vi "Car Data.vi"(1 "file path (dialog if empty)":path) -> (0 "CAR DATA":T1)   [LabVIEW 2014]
uses:
  Type Def/CAN Message.ctl
  Type Def/CAR Data Cluster.ctl
  <vilib>/Utility/file.llb/Read From Spreadsheet File (string).vi
panel:
  out "Time Size":i32
  out "number of rows":i32
  out "Time":dbl[](array[numeric]) format="%.2f"
  out "Array":T2[](array[typedef])
  out "DECAYIGN(+) - DECAYIGN(-)":dbl
  out "DECAYINJ(+) - DECAYINJ(-)":dbl
  out "DTPS-":dbl
  out "DTPS+":dbl
  out "Speed 2":dbl
  out "Speed 1":dbl
  out "Phase High":dbl
  out "Phase Low":dbl
  out "Spark 1":dbl
  out "Inj Low":dbl
  out "K Lambda 2":dbl
  out "K Lambda 1":dbl
  out "Lambda 2 AVG":dbl
  out "Lambda 2 RAW":dbl
  out "Lambda 1 RAW":dbl
  out "Lambda 1 AVG":dbl
  out "BAR0":u32
  out "VBB 3":dbl
  out "VBB 2":dbl
  out "VBB 1":dbl
  out "T Oil":u32
  out "T Air":i32
  out "T H20":i32
  out "map":u32
  out "TPS":dbl
  out "rev/min":u32
  out "revs":u32
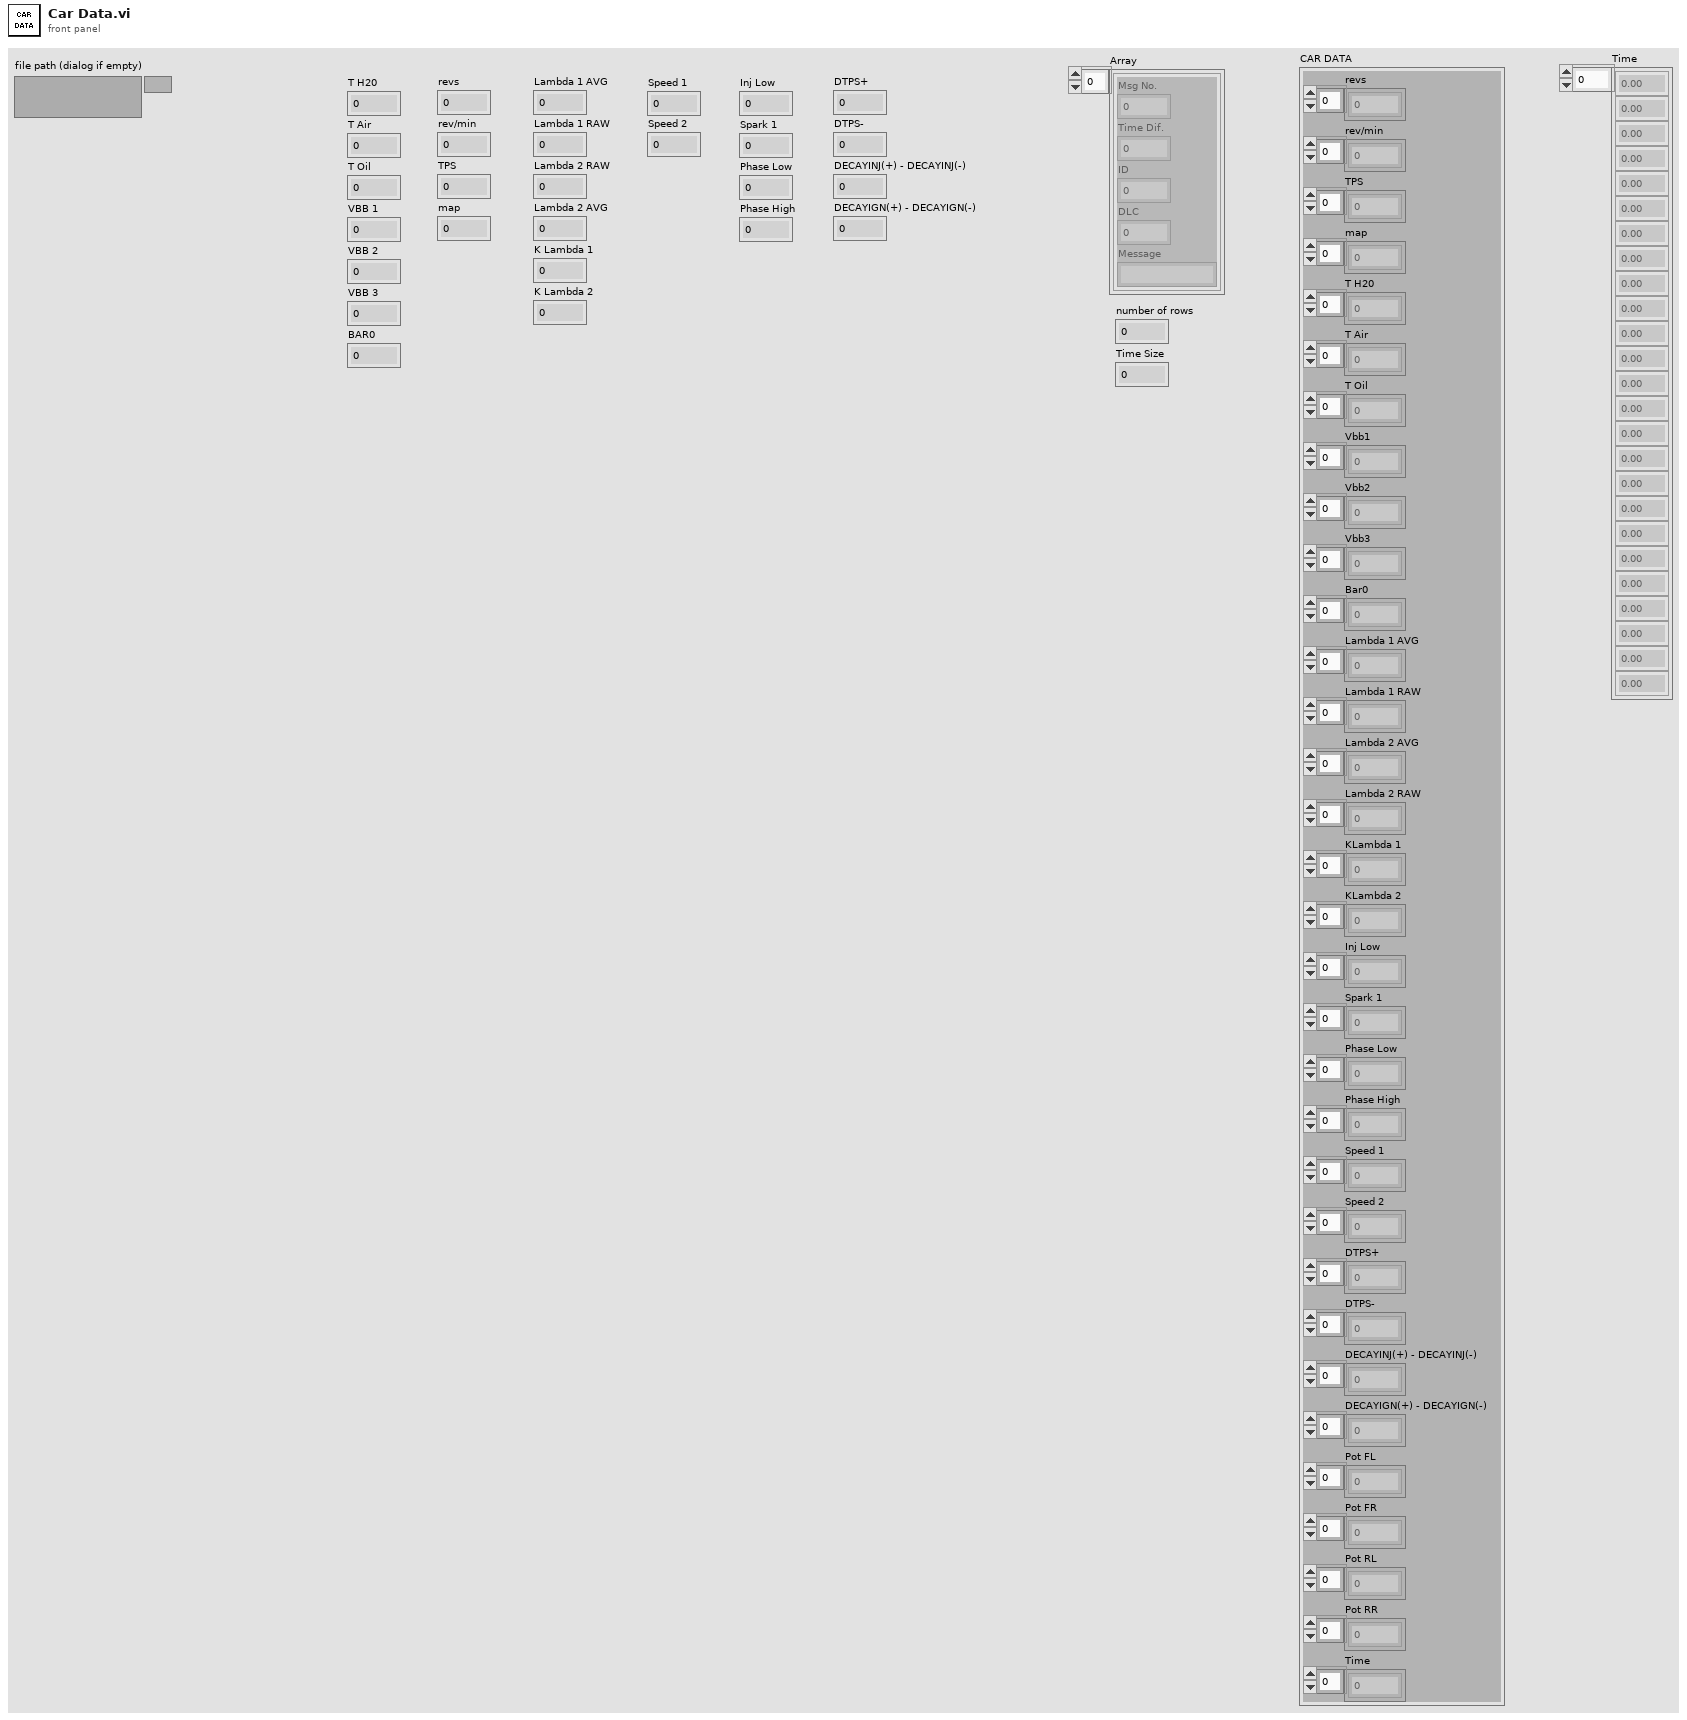
[diagram p1: front panel]
types:
  T1 = typedef "CAR Data Cluster.ctl" = cluster{"revs":dbl[], "rev/min":dbl[], "TPS":dbl[], "map":dbl[], "T H20":dbl[], "T Air":dbl[], "T Oil":dbl[], "Vbb1":dbl[], "Vbb2":dbl[], "Vbb3":dbl[], "Bar0":dbl[], "Lambda 1 AVG":dbl[], "Lambda 1 RAW":dbl[], "Lambda 2 AVG":dbl[], "Lambda 2 RAW":dbl[], "KLambda 1":dbl[], "KLambda 2":dbl[], "Inj Low":dbl[], "Spark 1":dbl[], "Phase Low":dbl[], "Phase High":dbl[], "Speed 1":dbl[], "Speed 2":dbl[], "DTPS+":dbl[], "DTPS-":dbl[], "DECAYINJ(+) - DECAYINJ(-)":dbl[], "DECAYIGN(+) - DECAYIGN(-)":dbl[], "Pot FL":dbl[], "Pot FR":dbl[], "Pot RL":dbl[], "Pot RR":dbl[], "Time":dbl[]}
  T2 = typedef "CAN Message.ctl" = cluster{"Msg No.":i32, "Time Dif.":i32, "ID":i32, "DLC":i32, "Message":string}
  T3 = cluster{"revs":dbl[], "rev/min":dbl[], "TPS":dbl[], "map":dbl[], "T H20":dbl[], "T Air":dbl[], "T Oil":dbl[], "Vbb1":dbl[], "Vbb2":dbl[], "Vbb3":dbl[], "Bar0":dbl[], "Lambda 1 AVG":dbl[], "Lambda 1 RAW":dbl[], "Lambda 2 AVG":dbl[], "Lambda 2 RAW":dbl[], "KLambda 1":dbl[], "KLambda 2":dbl[], "Inj Low":dbl[], "Spark 1":dbl[], "Phase Low":dbl[], "Phase High":dbl[], "Speed 1":dbl[], "Speed 2":dbl[], "DTPS+":dbl[], "DTPS-":dbl[], "DECAYINJ(+) - DECAYINJ(-)":dbl[], "DECAYIGN(+) - DECAYIGN(-)":dbl[], "Pot FL":dbl[], "Pot FR":dbl[], "Pot RL":dbl[], "Pot RR":dbl[], "Time":dbl[]}
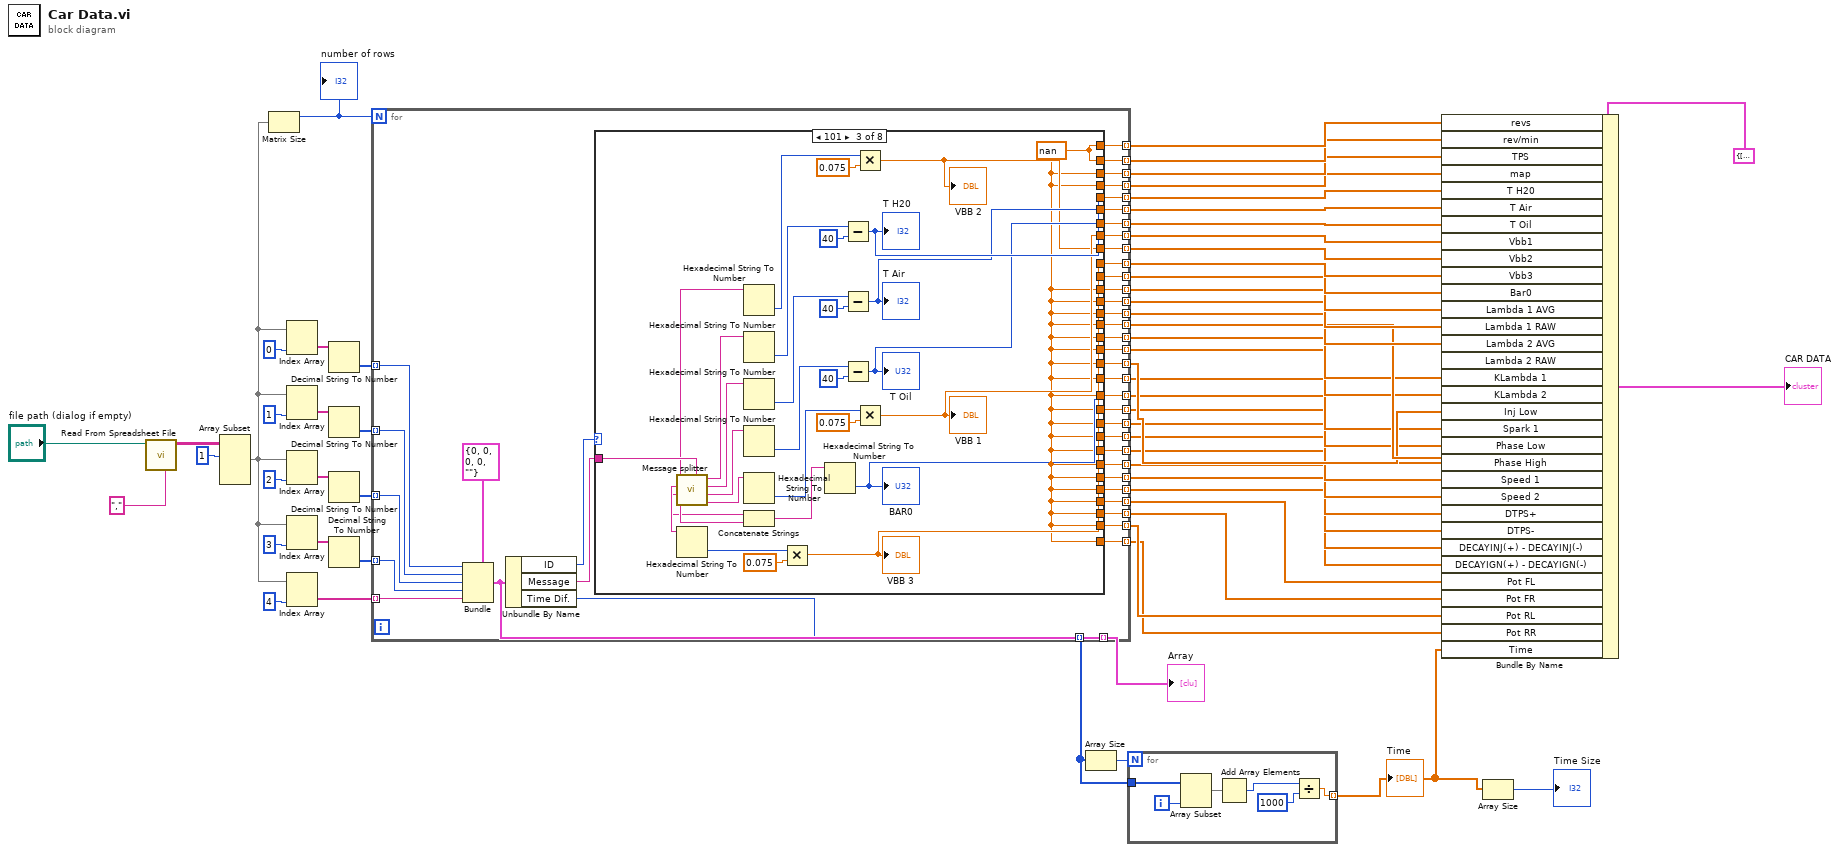
[diagram p0: block diagram]
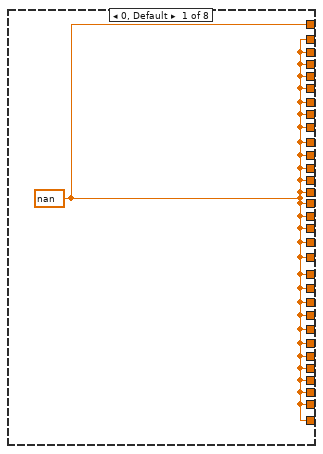
[diagram p2: hidden frame]
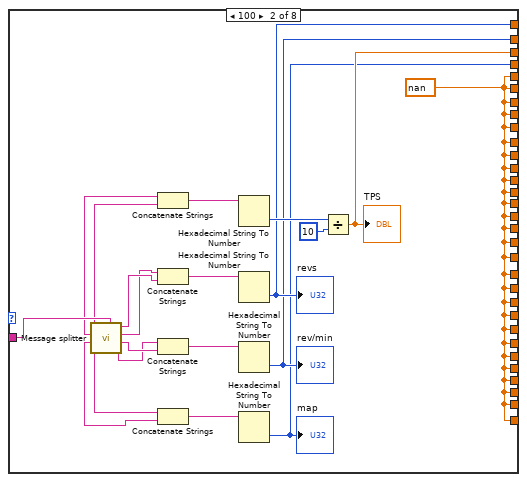
[diagram p3: hidden frame]
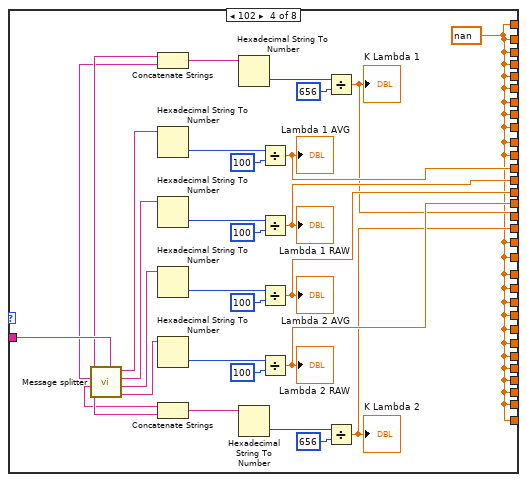
[diagram p4: hidden frame]
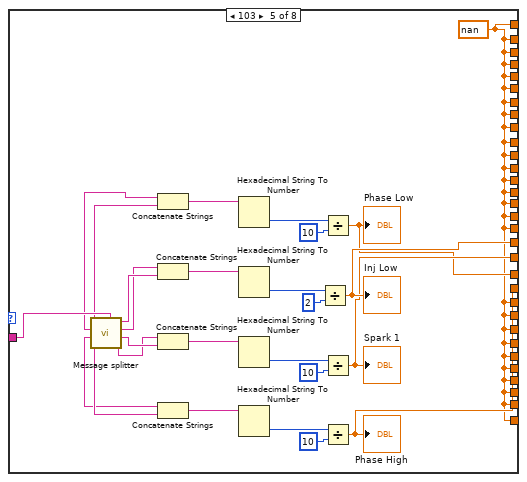
[diagram p5: hidden frame]
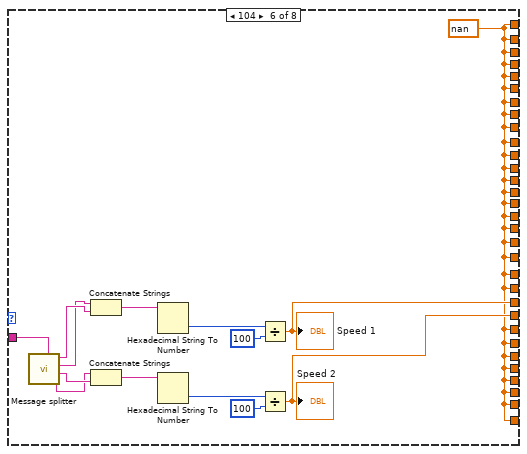
[diagram p6: hidden frame]
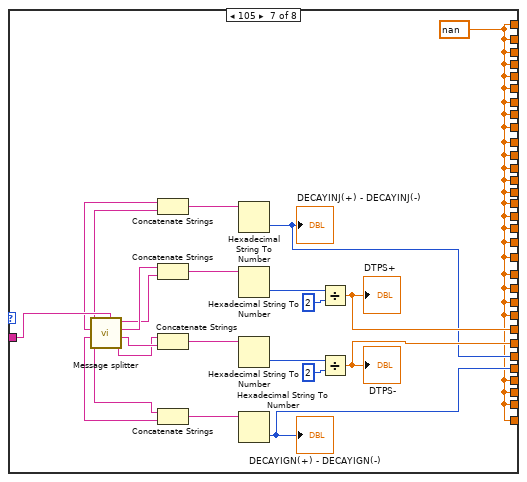
[diagram p7: hidden frame]
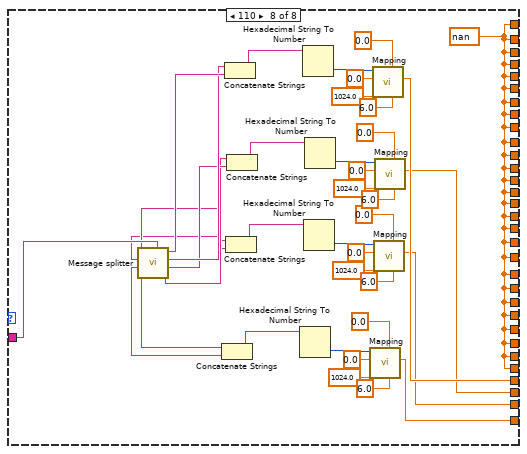
[diagram p8: hidden frame]
diagram:
  n1 = call-poly <vilib>:"Read From Spreadsheet File.vi"("delimiter (\\t)"="," ("delimiter (\\t)"), "file path (dialog if empty)"="file path (dialog if empty)") -> ("all rows"=w40:string[][])  [unwired: 5 in, 4 out]
  n2 = Array Subset(array=w40, index (row)=1 ("index")) -> (w51:string[][])  [unwired: 3 in]
  n3 = Matrix Size(0:w51) -> (1:w56:i32)  [unwired: 1 out]
  "number of rows" <- w56
  n4 = Index Array(array=w51, index (col)=0 ("index")) -> (element=w45:string[])  [unwired: 1 in]
  n5 = Index Array(array=w51, index (col)=1 ("index")) -> (element=w44:string[])  [unwired: 1 in]
  n6 = Index Array(array=w51, index (col)=2 ("index")) -> (element=w43:string[])  [unwired: 1 in]
  n7 = Index Array(array=w51, index (col)=3 ("index")) -> (element=w42:string[])  [unwired: 1 in]
  n8 = Index Array(array=w51, index (col)=4 ("index")) -> (element=w41:string[])  [unwired: 1 in]
  n9 = Decimal String To Number(string=w45) -> (number=w55:i32[])  [unwired: 2 in, 1 out]
  n10 = Decimal String To Number(string=w44) -> (number=w54:i32[])  [unwired: 2 in, 1 out]
  n11 = Decimal String To Number(string=w43) -> (number=w53:i32[])  [unwired: 2 in, 1 out]
  n12 = Decimal String To Number(string=w42) -> (number=w52:i32[])  [unwired: 2 in, 1 out]
  n13 = for {
    N: w56 -> [_]
    tunnel: w55 -> [w98] mode=indexing
    tunnel: w54 -> [w97] mode=indexing
    tunnel: w53 -> [w96] mode=indexing
    tunnel: w52 -> [w95] mode=indexing
    tunnel: [w93] -> w37 mode=indexing
    tunnel: w41 -> [w94] mode=indexing
    tunnel: [w90] -> w39 mode=indexing
    tunnel: [w89] -> w33 mode=indexing
    tunnel: [w88] -> w35 mode=indexing
    tunnel: [w87] -> w34 mode=indexing
    tunnel: [w86] -> w32 mode=indexing
    tunnel: [w85] -> w31 mode=indexing
    tunnel: [w84] -> w30 mode=indexing
    tunnel: [w83] -> w29 mode=indexing
    tunnel: [w82] -> w28 mode=indexing
    tunnel: [w81] -> w27 mode=indexing
    tunnel: [w80] -> w26 mode=indexing
    tunnel: [w79] -> w25 mode=indexing
    tunnel: [w78] -> w24 mode=indexing
    tunnel: [w77] -> w23 mode=indexing
    tunnel: [w76] -> w22 mode=indexing
    tunnel: [w75] -> w21 mode=indexing
    tunnel: [w74] -> w20 mode=indexing
    tunnel: [w73] -> w19 mode=indexing
    tunnel: [w72] -> w18 mode=indexing
    tunnel: [w71] -> w17 mode=indexing
    tunnel: [w70] -> w16 mode=indexing
    tunnel: [w69] -> w15 mode=indexing
    tunnel: [w68] -> w14 mode=indexing
    tunnel: [w67] -> w13 mode=indexing
    tunnel: [w66] -> w12 mode=indexing
    tunnel: [w65] -> w11 mode=indexing
    tunnel: [w64] -> w10 mode=indexing
    tunnel: [w63] -> w9 mode=indexing
    tunnel: [w62] -> w7 mode=indexing
    tunnel: [w61] -> w6 mode=indexing
    tunnel: [w60] -> w5 mode=indexing
    tunnel: [w59] -> w4 mode=indexing
    n14 = Bundle(cluster=T2 {"Msg No."=0, "Time Dif."=0, "ID"=0, "DLC"=0, "Message"=""}, "Msg No."=w98, "Time Dif."=w97, "ID"=w96, "DLC"=w95, "Message"=w94) -> (w93:T2)
    n15 = Unbundle By Name(w93) -> ("ID"=w92:i32, "Message"=w91:string, "Time Dif."=w90:i32)
    n16 = case shown="101" w92 {
      tunnel: w91 -> [_ w114 w137 w180 w206 w220 w242 w280]
      tunnel: [w100 w113 w121 w151 w181 w207 w221 w279] -> w89
      tunnel: [w100 w112 w121 w151 w181 w207 w221 w279] -> w88
      tunnel: [w100 w111 w121 w151 w181 w207 w221 w279] -> w87
      tunnel: [w100 w110 w121 w151 w181 w207 w221 w279] -> w86
      tunnel: [w100 w101 w130 w151 w181 w207 w221 w279] -> w85
      tunnel: [w100 w101 w129 w151 w181 w207 w221 w279] -> w84
      tunnel: [w100 w101 w128 w151 w181 w207 w221 w279] -> w83
      tunnel: [w100 w101 w127 w151 w181 w207 w221 w279] -> w82
      tunnel: [w100 w101 w126 w151 w181 w207 w221 w279] -> w81
      tunnel: [w100 w101 w125 w151 w181 w207 w221 w279] -> w80
      tunnel: [w100 w101 w124 w151 w181 w207 w221 w279] -> w79
      tunnel: [w100 w101 w121 w159 w181 w207 w221 w279] -> w78
      tunnel: [w100 w101 w121 w158 w181 w207 w221 w279] -> w77
      tunnel: [w100 w101 w121 w157 w181 w207 w221 w279] -> w76
      tunnel: [w100 w101 w121 w156 w181 w207 w221 w279] -> w75
      tunnel: [w100 w101 w121 w155 w181 w207 w221 w279] -> w74
      tunnel: [w100 w101 w121 w154 w181 w207 w221 w279] -> w73
      tunnel: [w100 w101 w121 w151 w193 w207 w221 w279] -> w72
      tunnel: [w100 w101 w121 w151 w192 w207 w221 w279] -> w71
      tunnel: [w100 w101 w121 w151 w191 w207 w221 w279] -> w70
      tunnel: [w100 w101 w121 w151 w190 w207 w221 w279] -> w69
      tunnel: [w100 w101 w121 w151 w181 w213 w221 w279] -> w68
      tunnel: [w100 w101 w121 w151 w181 w212 w221 w279] -> w67
      tunnel: [w100 w101 w121 w151 w181 w207 w233 w279] -> w66
      tunnel: [w100 w101 w121 w151 w181 w207 w232 w279] -> w65
      tunnel: [w100 w101 w121 w151 w181 w207 w231 w279] -> w64
      tunnel: [w100 w101 w121 w151 w181 w207 w230 w279] -> w63
      tunnel: [w100 w101 w121 w151 w181 w207 w221 w270] -> w62
      tunnel: [w100 w101 w121 w151 w181 w207 w221 w261] -> w61
      tunnel: [w100 w101 w121 w151 w181 w207 w221 w244] -> w60
      tunnel: [w100 w101 w121 w151 w181 w207 w221 w243] -> w59
      frame 0, Default {
        w100 = nan
      }
      frame 100 {
        w101 = nan
        n17 = call "Message splitter.vi"("Message in"=w114) -> ("Byte 4"=w104:string, "Byte 3"=w105:string, "Byte 2"=w106:string, "Byte 1"=w107:string, "Byte 8"=w102:string, "Byte 7"=w103:string, "Byte 6"=w109:string, "Byte 5"=w108:string)  [unwired: 3 in]
        n18 = Concatenate Strings(w109, w108) -> (w118:string)
        n19 = Concatenate Strings(w106, w107) -> (w120:string)
        n20 = Concatenate Strings(w104, w105) -> (w119:string)
        n21 = Concatenate Strings(w102, w103) -> (w115:string)
        n22 = Hexadecimal String To Number(string=w118) -> (number=w117:u32)  [unwired: 2 in, 1 out]
        n23 = Hexadecimal String To Number(string=w120) -> (number=w112:u32)  [unwired: 2 in, 1 out]
        "revs" <- w112
        n24 = Hexadecimal String To Number(string=w119) -> (number=w111:u32)  [unwired: 2 in, 1 out]
        "rev/min" <- w111
        n25 = Hexadecimal String To Number(string=w115) -> (number=w110:u32)  [unwired: 2 in, 1 out]
        "map" <- w110
        n26 = Divide(x=w117, y=u32 10) -> (x/y=w113:dbl)
        "TPS" <- w113
      }
      frame 101 {
        w121 = nan
        n27 = call "Message splitter.vi"("Message in"=w137) -> ("Byte 4"=w133:string, "Byte 3"=w134:string, "Byte 2"=w135:string, "Byte 1"=w136:string, "Byte 8"=w123:string, "Byte 7"=w122:string, "Byte 6"=w131:string, "Byte 5"=w132:string)  [unwired: 3 in]
        n28 = Hexadecimal String To Number(string=w131) -> (number=w140:u32)  [unwired: 2 in, 1 out]
        n29 = Hexadecimal String To Number(string=w132) -> (number=w142:u32)  [unwired: 2 in, 1 out]
        n30 = Hexadecimal String To Number(string=w136) -> (number=w150:u32)  [unwired: 2 in, 1 out]
        n31 = Hexadecimal String To Number(string=w135) -> (number=w147:u32)  [unwired: 2 in, 1 out]
        n32 = Hexadecimal String To Number(string=w134) -> (number=w145:u32)  [unwired: 2 in, 1 out]
        n33 = Hexadecimal String To Number(string=w133) -> (number=w144:u32)  [unwired: 2 in, 1 out]
        n34 = Concatenate Strings(w122, w123) -> (w138:string)
        n35 = Multiply(x=w140, y=0.075) -> (x*y=w125:dbl)
        "VBB 3" <- w125
        n36 = Hexadecimal String To Number(string=w138) -> (number=w124:u32)  [unwired: 2 in, 1 out]
        "BAR0" <- w124
        n37 = Subtract(x=w150, y=u32 40) -> (x-y=w130:u32)
        "T H20" <- w130
        n38 = Subtract(x=w147, y=u32 40) -> (x-y=w129:u32)
        "T Air" <- w129
        n39 = Subtract(x=w145, y=u32 40) -> (x-y=w128:u32)
        "T Oil" <- w128
        n40 = Multiply(x=w142, y=0.075) -> (x*y=w126:dbl)
        "VBB 2" <- w126
        n41 = Multiply(x=w144, y=0.075) -> (x*y=w127:dbl)
        "VBB 1" <- w127
      }
      frame 102 {
        w151 = nan
        n42 = call "Message splitter.vi"("Message in"=w180) -> ("Byte 4"=w168:string, "Byte 3"=w169:string, "Byte 2"=w170:string, "Byte 1"=w179:string, "Byte 8"=w153:string, "Byte 7"=w152:string, "Byte 6"=w166:string, "Byte 5"=w167:string)  [unwired: 3 in]
        n43 = Concatenate Strings(w167, w166) -> (w163:string)
        n44 = Hexadecimal String To Number(string=w179) -> (number=w178:u32)  [unwired: 2 in, 1 out]
        n45 = Hexadecimal String To Number(string=w170) -> (number=w176:u32)  [unwired: 2 in, 1 out]
        n46 = Hexadecimal String To Number(string=w169) -> (number=w172:u32)  [unwired: 2 in, 1 out]
        n47 = Hexadecimal String To Number(string=w168) -> (number=w174:u32)  [unwired: 2 in, 1 out]
        n48 = Concatenate Strings(w152, w153) -> (w160:string)
        n49 = Hexadecimal String To Number(string=w163) -> (number=w165:u32)  [unwired: 2 in, 1 out]
        n50 = Hexadecimal String To Number(string=w160) -> (number=w162:u32)  [unwired: 2 in, 1 out]
        n51 = Divide(x=w178, y=u32 100) -> (x/y=w159:dbl)
        "Lambda 1 AVG" <- w159
        n52 = Divide(x=w176, y=u32 100) -> (x/y=w158:dbl)
        "Lambda 1 RAW" <- w158
        n53 = Divide(x=w172, y=u32 100) -> (x/y=w157:dbl)
        "Lambda 2 AVG" <- w157
        n54 = Divide(x=w174, y=u32 100) -> (x/y=w156:dbl)
        "Lambda 2 RAW" <- w156
        n55 = Divide(x=w165, y=u32 656) -> (x/y=w155:dbl)
        "K Lambda 1" <- w155
        n56 = Divide(x=w162, y=u32 656) -> (x/y=w154:dbl)
        "K Lambda 2" <- w154
      }
      frame 103 {
        w181 = nan
        n57 = call "Message splitter.vi"("Message in"=w206) -> ("Byte 4"=w186:string, "Byte 3"=w187:string, "Byte 2"=w188:string, "Byte 1"=w189:string, "Byte 8"=w183:string, "Byte 7"=w182:string, "Byte 6"=w185:string, "Byte 5"=w184:string)  [unwired: 3 in]
        n58 = Concatenate Strings(w185, w184) -> (w199:string)
        n59 = Concatenate Strings(w188, w189) -> (w205:string)
        n60 = Concatenate Strings(w186, w187) -> (w202:string)
        n61 = Concatenate Strings(w182, w183) -> (w196:string)
        n62 = Hexadecimal String To Number(string=w199) -> (number=w198:u32)  [unwired: 2 in, 1 out]
        n63 = Hexadecimal String To Number(string=w205) -> (number=w204:u32)  [unwired: 2 in, 1 out]
        n64 = Hexadecimal String To Number(string=w202) -> (number=w201:u32)  [unwired: 2 in, 1 out]
        n65 = Hexadecimal String To Number(string=w196) -> (number=w195:u32)  [unwired: 2 in, 1 out]
        n66 = Divide(x=w204, y=u32 2) -> (x/y=w193:dbl)
        "Inj Low" <- w193
        n67 = Divide(x=w198, y=u32 10) -> (x/y=w191:dbl)
        "Phase Low" <- w191
        n68 = Divide(x=w201, y=u32 10) -> (x/y=w192:dbl)
        "Spark 1" <- w192
        n69 = Divide(x=w195, y=u32 10) -> (x/y=w190:dbl)
        "Phase High" <- w190
      }
      frame 104 {
        w207 = nan
        n70 = call "Message splitter.vi"("Message in"=w220) -> ("Byte 4"=w208:string, "Byte 3"=w209:string, "Byte 2"=w210:string, "Byte 1"=w211:string)  [unwired: 3 in, 4 out]
        n71 = Concatenate Strings(w210, w211) -> (w219:string)
        n72 = Concatenate Strings(w208, w209) -> (w214:string)
        n73 = Hexadecimal String To Number(string=w219) -> (number=w218:u32)  [unwired: 2 in, 1 out]
        n74 = Hexadecimal String To Number(string=w214) -> (number=w216:u32)  [unwired: 2 in, 1 out]
        n75 = Divide(x=w218, y=u32 100) -> (x/y=w213:dbl)
        "Speed 1" <- w213
        n76 = Divide(x=w216, y=u32 100) -> (x/y=w212:dbl)
        "Speed 2" <- w212
      }
      frame 105 {
        w221 = nan
        n77 = call "Message splitter.vi"("Message in"=w242) -> ("Byte 4"=w226:string, "Byte 3"=w227:string, "Byte 2"=w229:string, "Byte 1"=w228:string, "Byte 8"=w223:string, "Byte 7"=w222:string, "Byte 6"=w224:string, "Byte 5"=w225:string)  [unwired: 3 in]
        n78 = Concatenate Strings(w224, w225) -> (w235:string)
        n79 = Concatenate Strings(w229, w228) -> (w241:string)
        n80 = Concatenate Strings(w226, w227) -> (w238:string)
        n81 = Concatenate Strings(w223, w222) -> (w234:string)
        n82 = Hexadecimal String To Number(string=w235) -> (number=w231:u32)  [unwired: 2 in, 1 out]
        "DECAYINJ(+) - DECAYINJ(-)" <- w231
        n83 = Hexadecimal String To Number(string=w241) -> (number=w240:u32)  [unwired: 2 in, 1 out]
        n84 = Hexadecimal String To Number(string=w238) -> (number=w237:u32)  [unwired: 2 in, 1 out]
        n85 = Hexadecimal String To Number(string=w234) -> (number=w230:u32)  [unwired: 2 in, 1 out]
        "DECAYIGN(+) - DECAYIGN(-)" <- w230
        n86 = Divide(x=w240, y=u32 2) -> (x/y=w233:dbl)
        "DTPS+" <- w233
        n87 = Divide(x=w237, y=u32 2) -> (x/y=w232:dbl)
        "DTPS-" <- w232
      }
      frame 110 {
        w279 = nan
        n88 = call "Message splitter.vi"("Message in"=w280) -> ("Byte 4"=w262:string, "Byte 3"=w263:string, "Byte 2"=w277:string, "Byte 1"=w278:string, "Byte 8"=w246:string, "Byte 7"=w245:string, "Byte 6"=w247:string, "Byte 5"=w248:string)  [unwired: 3 in]
        n89 = Concatenate Strings(w246, w245) -> (w254:string)
        n90 = Concatenate Strings(w277, w278) -> (w276:string)
        n91 = Concatenate Strings(w247, w248) -> (w260:string)
        n92 = Concatenate Strings(w262, w263) -> (w269:string)
        n93 = Hexadecimal String To Number(string=w254) -> (number=w253:u32)  [unwired: 2 in, 1 out]
        n94 = Hexadecimal String To Number(string=w276) -> (number=w275:u32)  [unwired: 2 in, 1 out]
        n95 = Hexadecimal String To Number(string=w260) -> (number=w259:u32)  [unwired: 2 in, 1 out]
        n96 = Hexadecimal String To Number(string=w269) -> (number=w268:u32)  [unwired: 2 in, 1 out]
        n97 = call "Mapping.vi"("out_max"=6.0, "out_min"=0.0, "in_max"=1024.0, "in_min"=0.0, "x"=w253) -> ("y"=w243:dbl)  [unwired: 6 in]
        n98 = call "Mapping.vi"("out_max"=6.0, "out_min"=0.0, "in_max"=1024.0, "in_min"=0.0, "x"=w275) -> ("y"=w270:dbl)  [unwired: 6 in]
        n99 = call "Mapping.vi"("out_max"=6.0, "out_min"=0.0, "in_max"=1024.0, "in_min"=0.0, "x"=w259) -> ("y"=w244:dbl)  [unwired: 6 in]
        n100 = call "Mapping.vi"("out_max"=6.0, "out_min"=0.0, "in_max"=1024.0, "in_min"=0.0, "x"=w268) -> ("y"=w261:dbl)  [unwired: 6 in]
      }
    }
  }
  "Array" <- w37
  n101 = Array Size(array=w39) -> (size(s)=w38:i32)
  n102 = for {
    N: w38 -> [_]
    tunnel: w39 -> [w286]
    tunnel: [w281] -> w2 mode=indexing
    i -> [w285]
    n103 = Array Subset(array=w286, length=w285) -> (w284:i32[])  [unwired: 1 in]
    n104 = Add Array Elements(numeric array=w284) -> (sum=w283:i32)
    n105 = Divide(x=w283, y=1000) -> (x/y=w281:dbl)
  }
  "Time" <- w2
  n106 = Bundle By Name(cluster=T3 {"revs"=[], "rev/min"=[], "TPS"=[], "map"=[], "T H20"=[], "T Air"=[], "T Oil"=[], "Vbb1"=[], "Vbb2"=[], "Vbb3"=[], "Bar0"=[], "Lambda 1 AVG"=[], "Lambda 1 RAW"=[], "Lambda 2 AVG"=[], "Lambda 2 RAW"=[], "KLambda 1"=[], "KLambda 2"=[], "Inj Low"=[], "Spark 1"=[], "Phase Low"=[], "Phase High"=[], "Speed 1"=[], "Speed 2"=[], "DTPS+"=[], "DTPS-"=[], "DECAYINJ(+) - DECAYINJ(-)"=[], "DECAYIGN(+) - DECAYIGN(-)"=[], "Pot FL"=[], "Pot FR"=[], "Pot RL"=[], "Pot RR"=[], "Time"=[]}, "revs"=w35, "rev/min"=w34, "TPS"=w33, "map"=w32, "T H20"=w31, "T Air"=w30, "T Oil"=w29, "Vbb1"=w28, "Vbb2"=w27, "Vbb3"=w26, "Bar0"=w25, "Lambda 1 AVG"=w24, "Lambda 1 RAW"=w23, "Lambda 2 AVG"=w22, "Lambda 2 RAW"=w21, "KLambda 1"=w20, "KLambda 2"=w19, "Inj Low"=w18, "Spark 1"=w17, "Phase Low"=w16, "Phase High"=w15, "Speed 1"=w14, "Speed 2"=w13, "DTPS+"=w12, "DTPS-"=w11, "DECAYINJ(+) - DECAYINJ(-)"=w10, "DECAYIGN(+) - DECAYIGN(-)"=w9, "Pot FL"=w7, "Pot FR"=w6, "Pot RL"=w5, "Pot RR"=w4, "Time"=w2) -> (→"CAR DATA":T3)
  n107 = Array Size(array=w2) -> (size(s)=→"Time Size":i32)
